vi "RichToFlatw4lvgrpc_Msg_ToClient_1.vi"(5 "OutputClusterType":T1, 11 "InputCluster":T2) -> (3 "OutputCluster":T1)   [LabVIEW 2019, in "Generated_server.lvlib"]
uses:
  Generated_server.lvlib
  w4lvgrpc_Msg_ToClient_1_Flat.ctl
  w4lvgrpc_Msg_ToClient_1.ctl
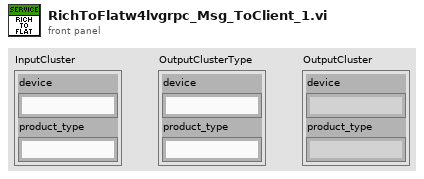
[diagram p1: front panel]
types:
  T1 = typedef "Generated_server.lvlib/w4lvgrpc_Msg_ToClient_1_Flat.ctl" = cluster{"device":string, "product_type":string}
  T2 = typedef "Generated_server.lvlib/w4lvgrpc_Msg_ToClient_1.ctl" = cluster{"device":string, "product_type":string}
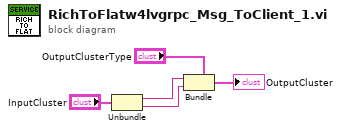
[diagram p0: block diagram]
diagram:
  n1 = Unbundle "Unbundle"("InputCluster") -> ("device"=w2:string, "product_type"=w1:string)
  n2 = Bundle "Bundle"(cluster="OutputClusterType", "device"=w2, "product_type"=w1) -> (→"OutputCluster":T1)
